vi "FindProxyObject.vi"(0 "remote ref":refnum<class "G#Object.lvclass">, 5 "error in (no error)":errorcluster) -> (14 "proxy ref":refnum<class "G#RemoteProxy.lvclass">, 17 "found":bool, 19 "error out":errorcluster)   [LabVIEW 2020, in "G#RemoteProxy.lvclass"]
doc: "Finds the proxy object."
uses:
  <vilib>/addons/_AddQ/G#Debugger/G#RemoteProxy/G#RemoteProxy.lvclass
  <vilib>/addons/_AddQ/G#Object/G#Object.lvclass
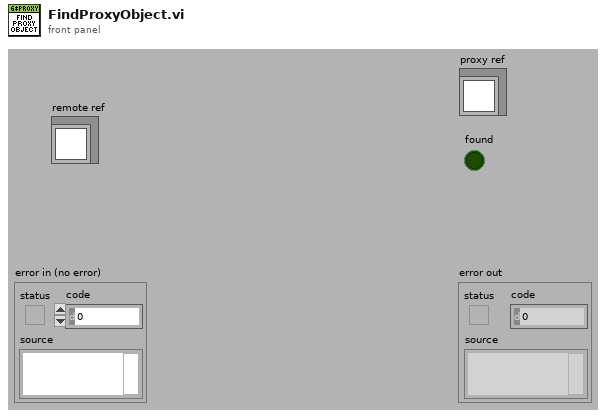
[diagram p1: front panel]
types:
  T1 = typedef "G#RemoteProxy.lvclass/ClassAttributesProxy.ctl" = cluster{"NoActiveProject":bool, "FullClassNames":string[], "FullClassPaths":path[], "RemoteRefs":refnum<class "G#Object.lvclass">[], "ProxyRefs":refnum<class "G#RemoteProxy.lvclass">[], "RemoteClassName":string[], "ProxyClassRefs":refnum<class "G#RemoteProxy.lvclass">[]}
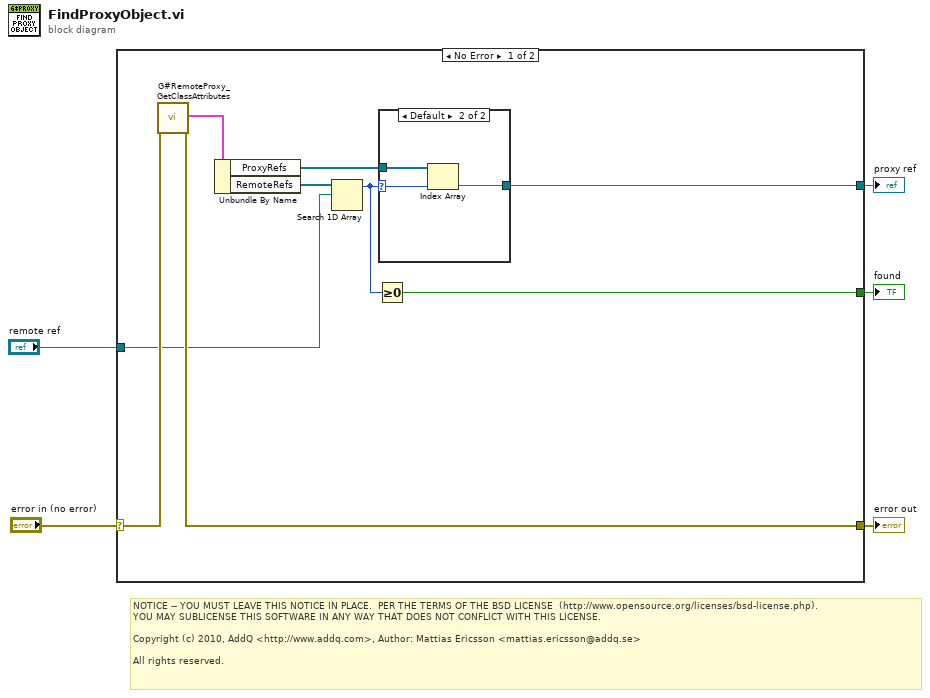
[diagram p0: block diagram]
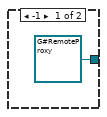
[diagram p2: hidden frame]
diagram:
  # "NOTICE -- YOU MUST LEAVE THIS NOTICE IN PLACE.  PER THE TERMS OF THE BSD LICENSE  (http://www.opensource.org/licenses/bsd-license.php).\nYOU MAY SUBLICENSE THIS SOFTWARE IN ANY WAY THAT DOES NOT CONFLICT WITH THIS LICENSE.\n\nCopyright (c) 2010, AddQ <http://www.addq.com>, Author: Mattias Ericsson <mattias.ericsson@addq.se>\n\nAll rights reserved."
  n1 = case shown="No Error" "error in (no error)" {
    selector: "error in (no error)" -> [w14 w19]
    tunnel: [w13 w19] -> w4
    tunnel: "remote ref" -> [w10 _]
    tunnel: [w8 _] -> w2
    tunnel: [w6 _] -> w1
    frame No Error {
      n2 = call <vilib>:"G#RemoteProxy_GetClassAttributes.vi"("error in (no error)"=w14) -> ("class attributes"=w12:T1, "error out"=w13:errorcluster)  [unwired: 15 in, 2 out]
      n3 = Unbundle By Name(w12) -> ("ProxyRefs"=w9:refnum<class "G#RemoteProxy.lvclass">[], "RemoteRefs"=w11:refnum<class "G#Object.lvclass">[])
      n4 = Search 1D Array(1D array=w11, element=w10) -> (index of element=w7:i32)  [unwired: 1 in]
      n5 = Greater Or Equal To 0?(x=w7) -> (x >= 0?=w6:bool)
      n6 = case shown="Default" w7 {
        selector: w7 -> [_ w17]
        tunnel: w9 -> [_ w18]
        tunnel: [refnum<class "G#RemoteProxy.lvclass"> refnum ("G#RemoteProxy.lvclass") w16] -> w8
        frame -1 {
        }
        frame Default {
          n7 = Index Array(array=w18, index=w17) -> (element=w16:refnum<class "G#RemoteProxy.lvclass">)
        }
      }
    }
    frame Error {
    }
  }
  "error out" <- w4
  "proxy ref" <- w2
  "found" <- w1
